vi "projekt.vi"() -> ()   [LabVIEW 2023]
doc: "Use this template to build a standard state machine design pattern. Each state executes code and determines which state to transition to. Contrast this design pattern with the User Interface Event Handler pattern, in which code executes in response to user actions. Contrast this design pattern also with the Queued Message Handler pattern, in which each message handling code can queue zero or more new messages.\nNote: This template does not contain the most recent programming guidelines recommended by National Instruments. For a complete, project-based implementation of the Standard State Machine pattern, use the Create Project dialog box instead of this template."
uses:
  projekt_stany.ctl
  <vilib>/DAQmx/read.llb/DAQmx Read (Digital 1D Bool 1Chan 1Samp).vi
  <vilib>/DAQmx/create/channels.llb/DAQmx Create Channel (DI-Digital Input).vi
  <vilib>/DAQmx/miscellaneous.llb/DAQmx Fill In Error Info.vi
panel:
  out "Nastepny Gracz":string
  in  "Wybierz Kto zaczyna":bool
  out "Wynik":string
  out "String 9":string
  out "String 8":string
  out "String 7":string
  out "String 6":string
  out "String 5":string
  out "String 4":string
  out "String 3":string
  out "String 2":string
  out "String":string
  in  "Stop":bool
  out "Kolumna":dbl
  out "Wiersz":dbl
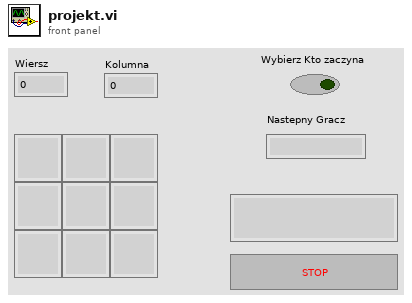
[diagram p1: front panel]
types:
  T1 = typedef "projekt_stany.ctl" = enum16{"Czysc", "Zapisz", "Wpisz", "Sprawdz", "Czytaj", "Initialize", "Stop"}
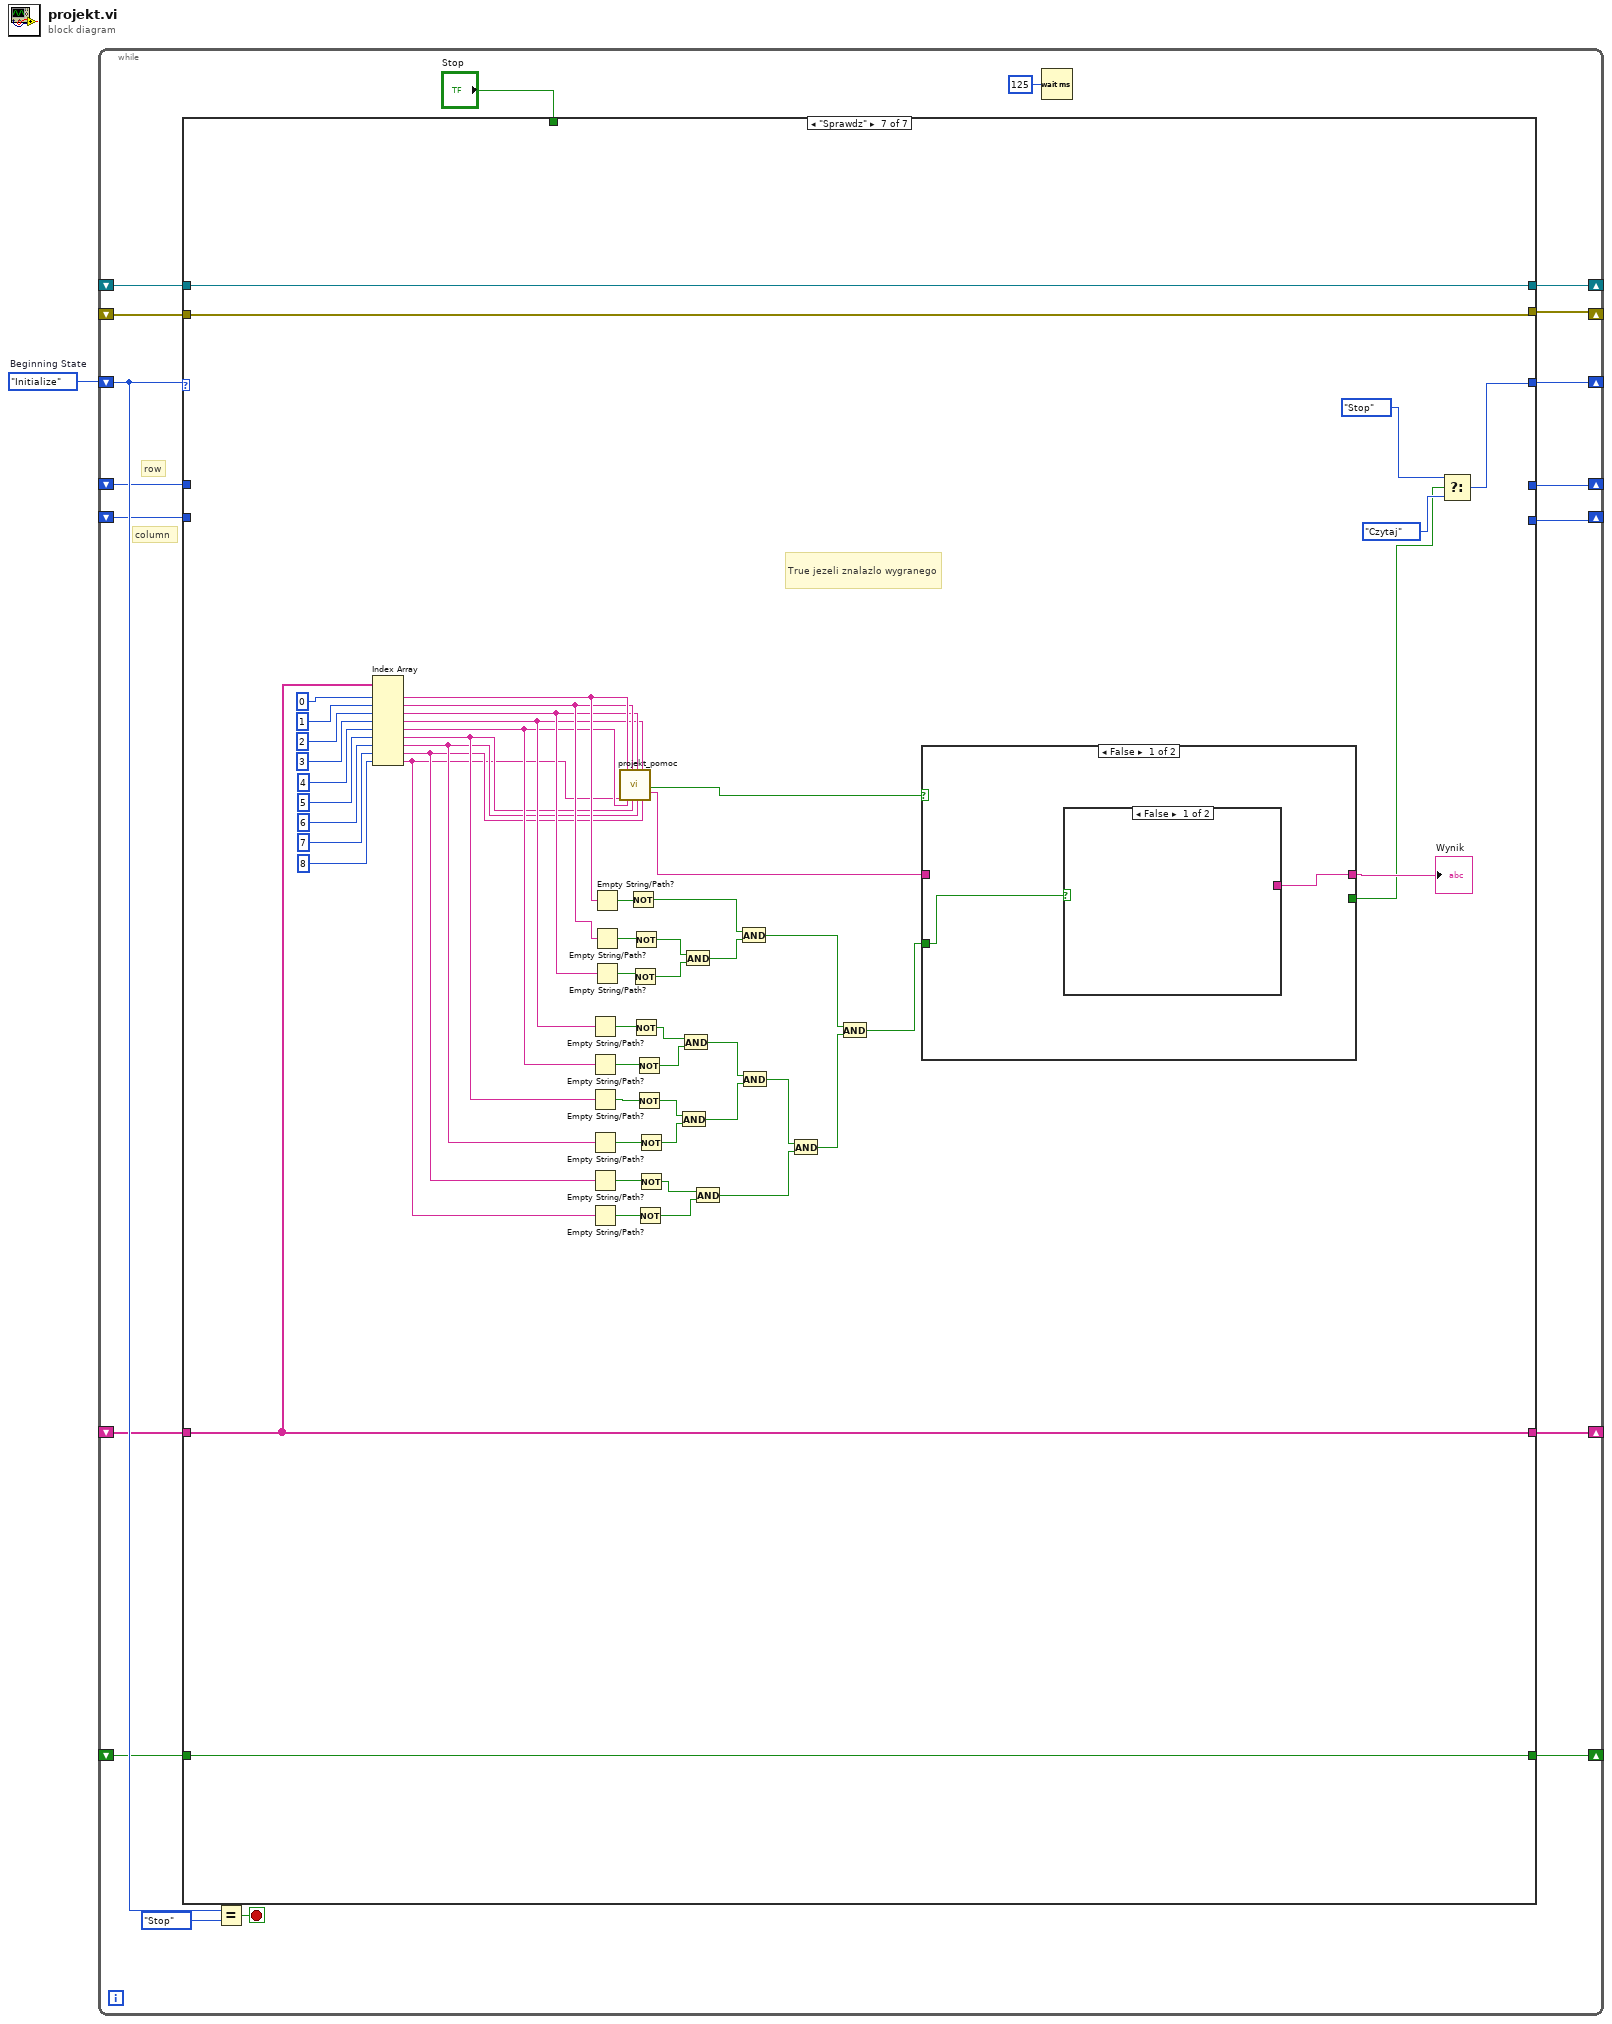
[diagram p0: block diagram]
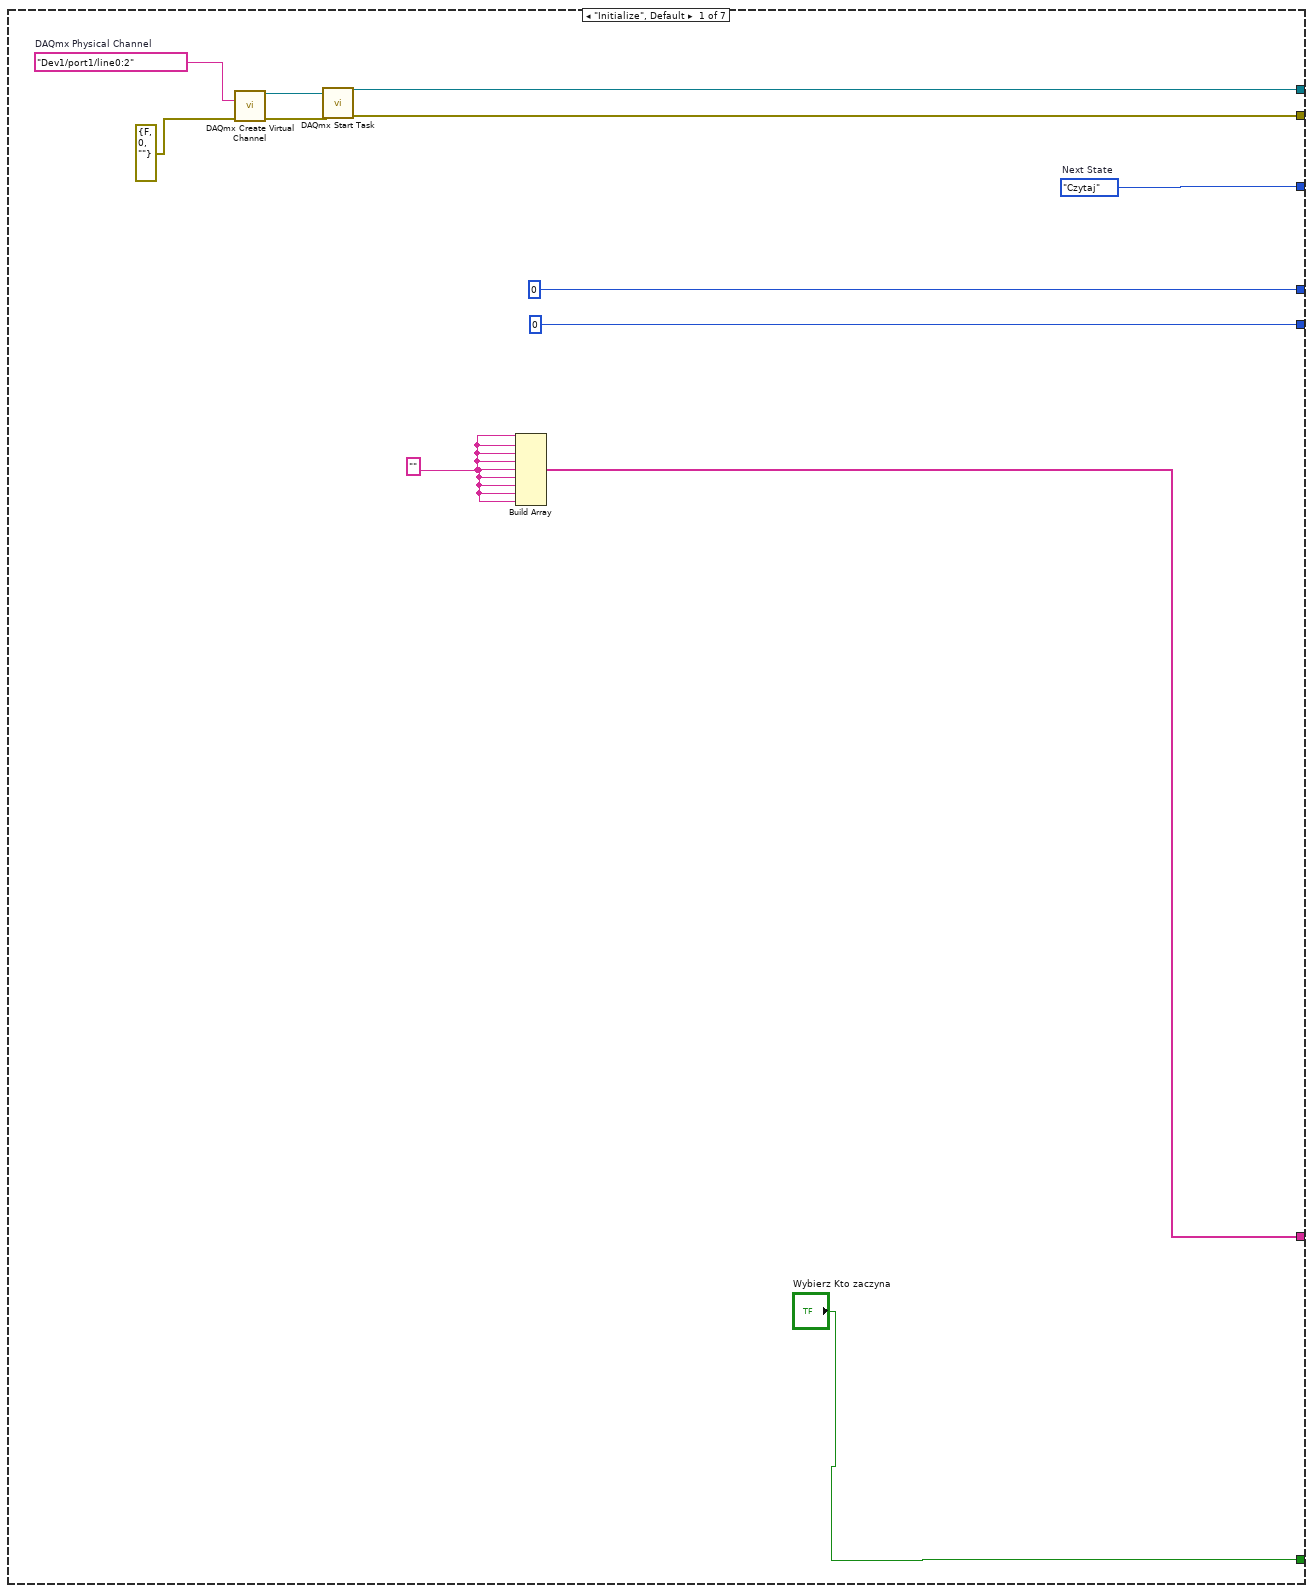
[diagram p2: hidden frame]
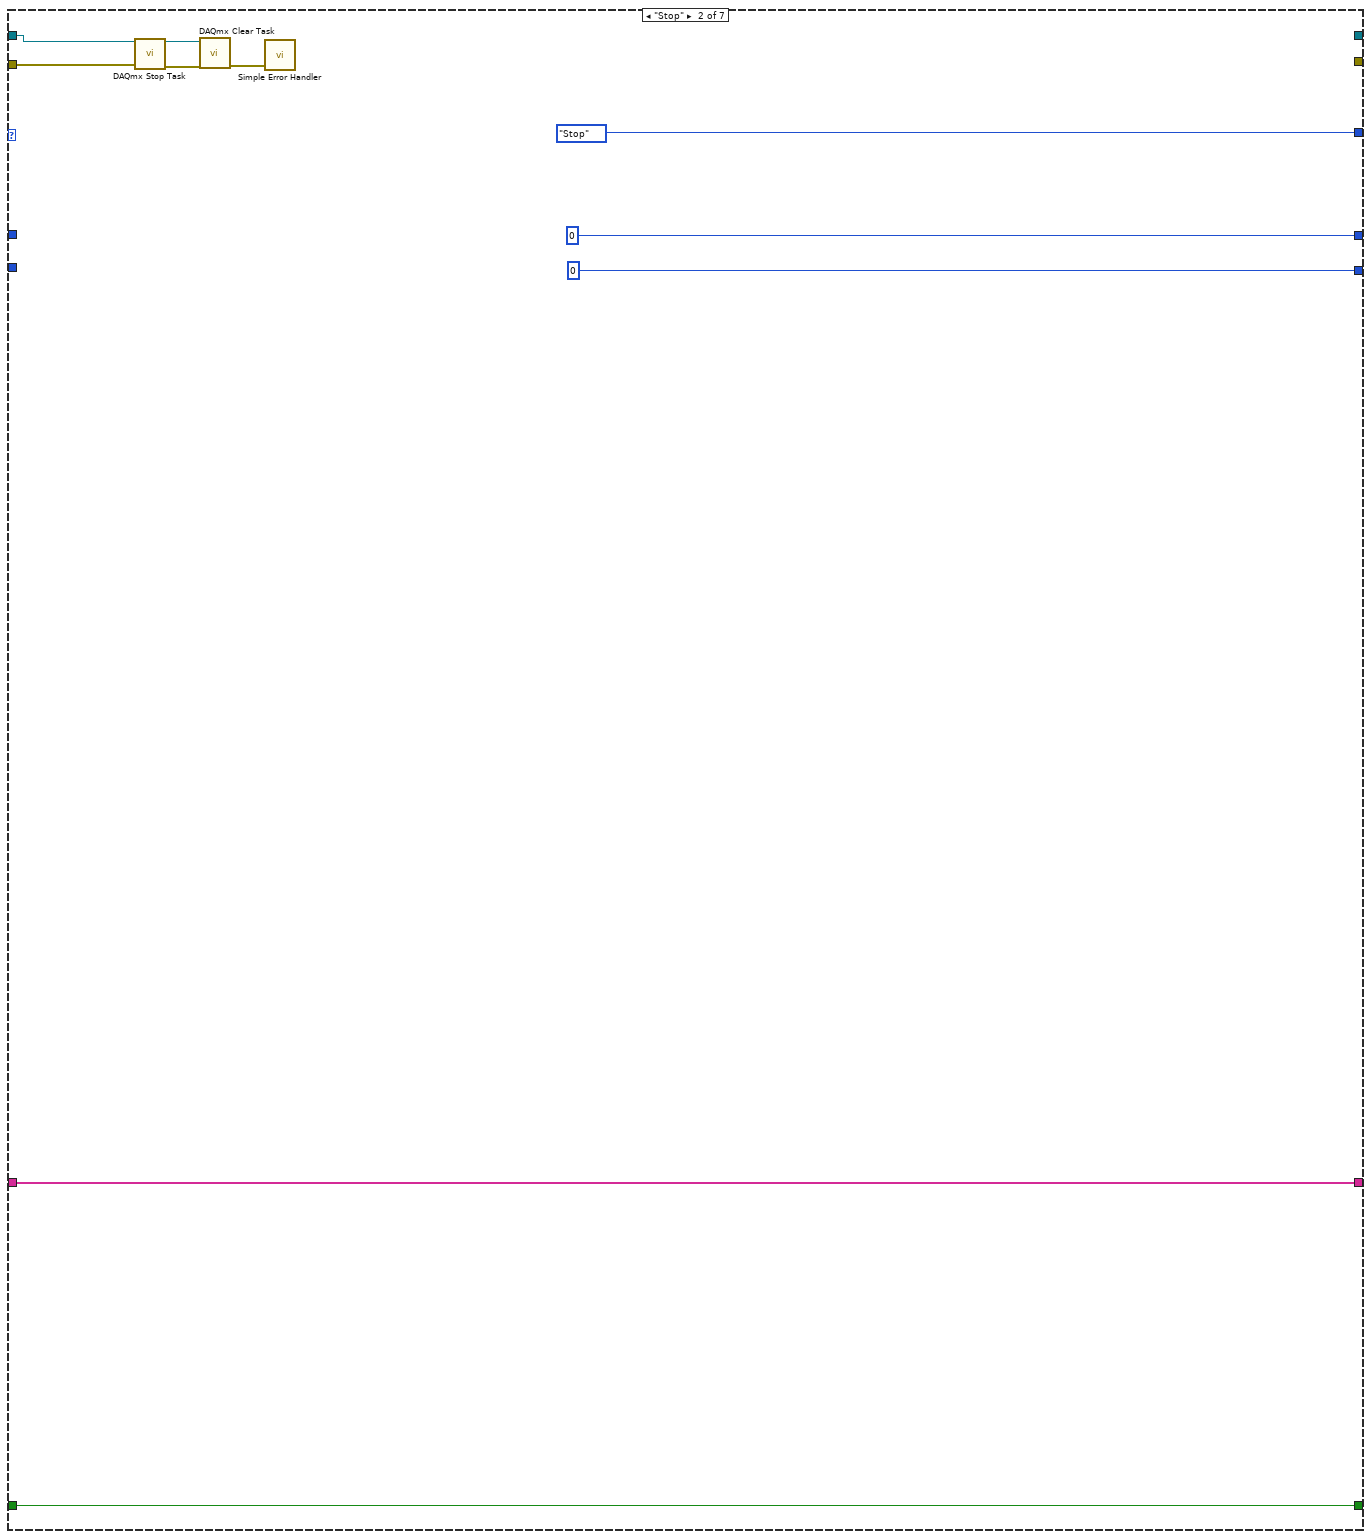
[diagram p3: hidden frame]
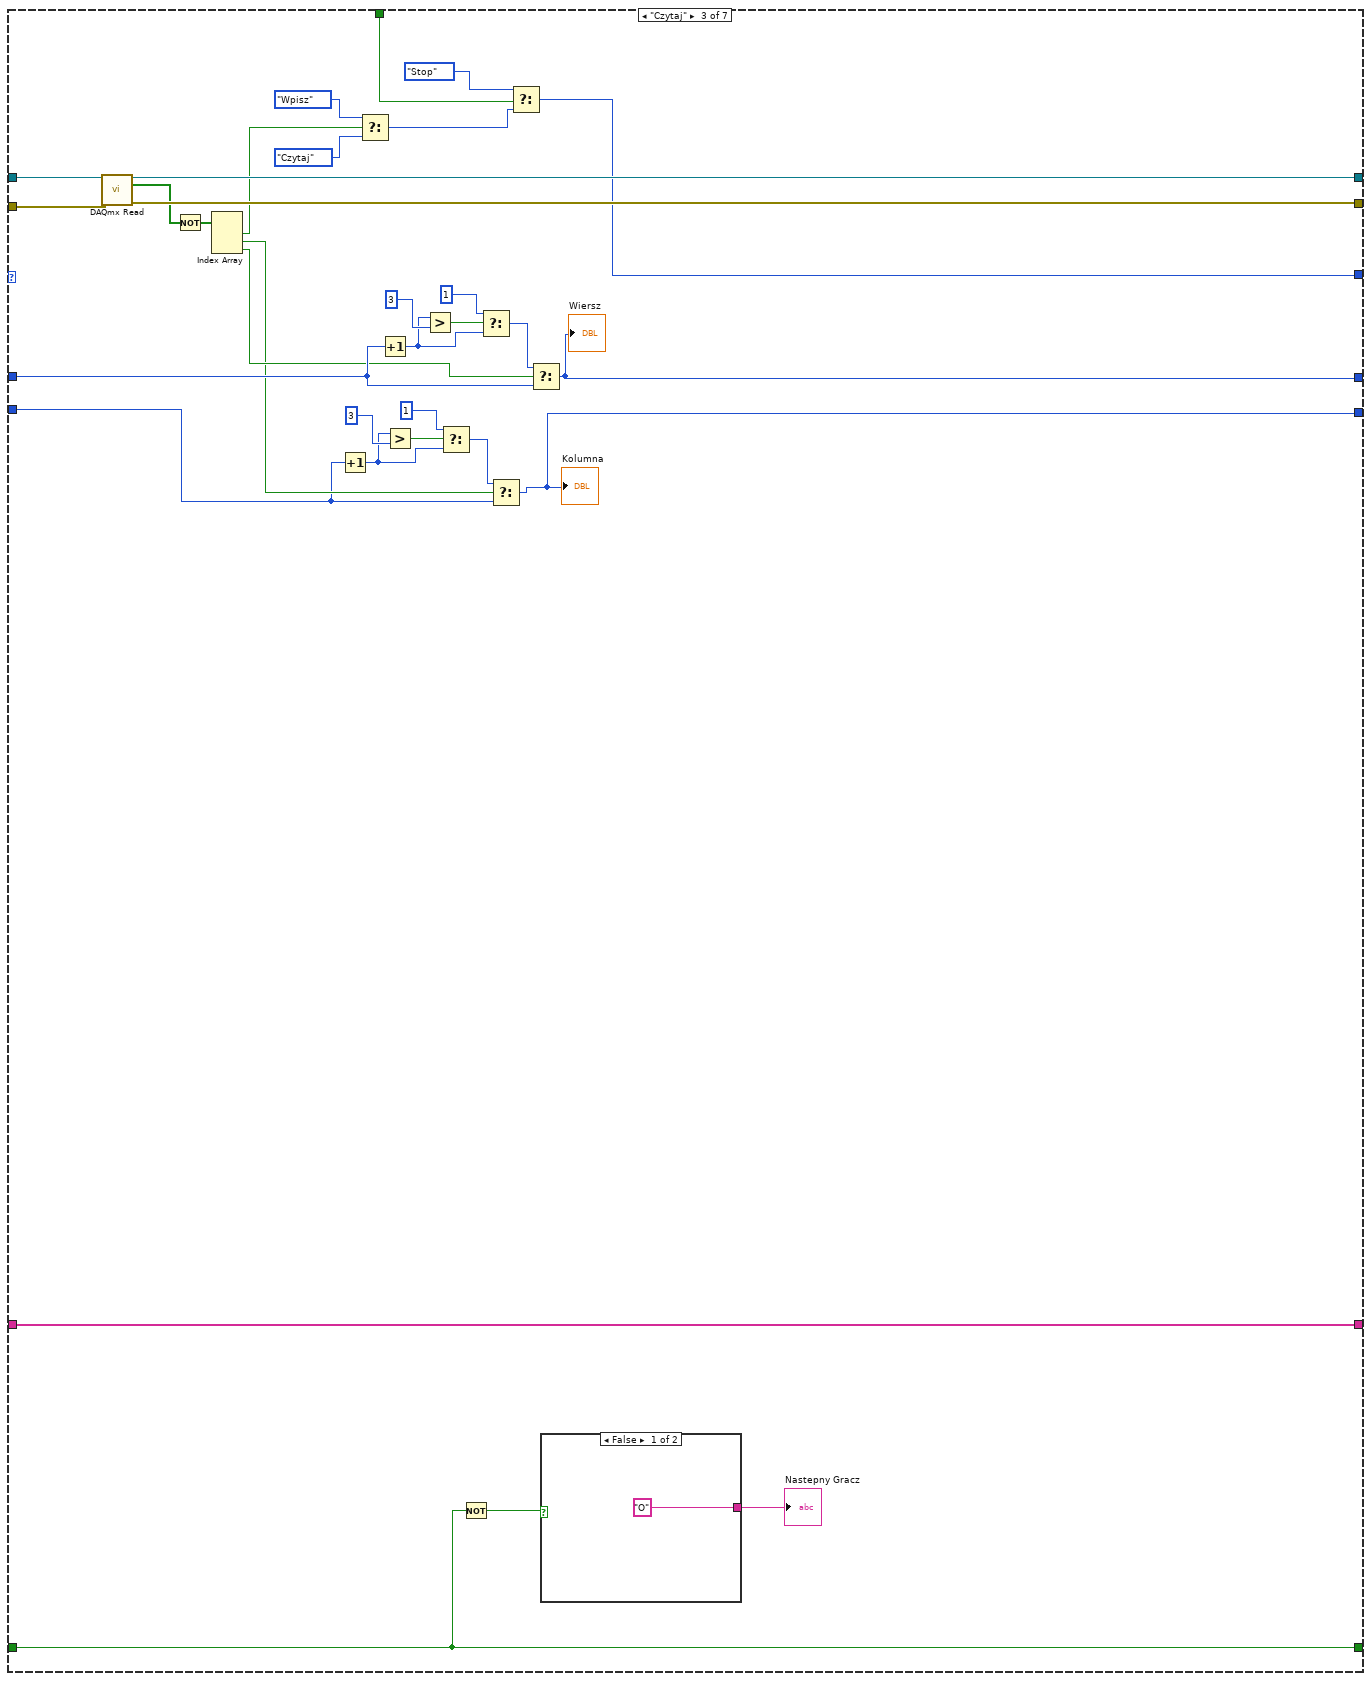
[diagram p4: hidden frame]
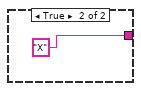
[diagram p5: hidden frame]
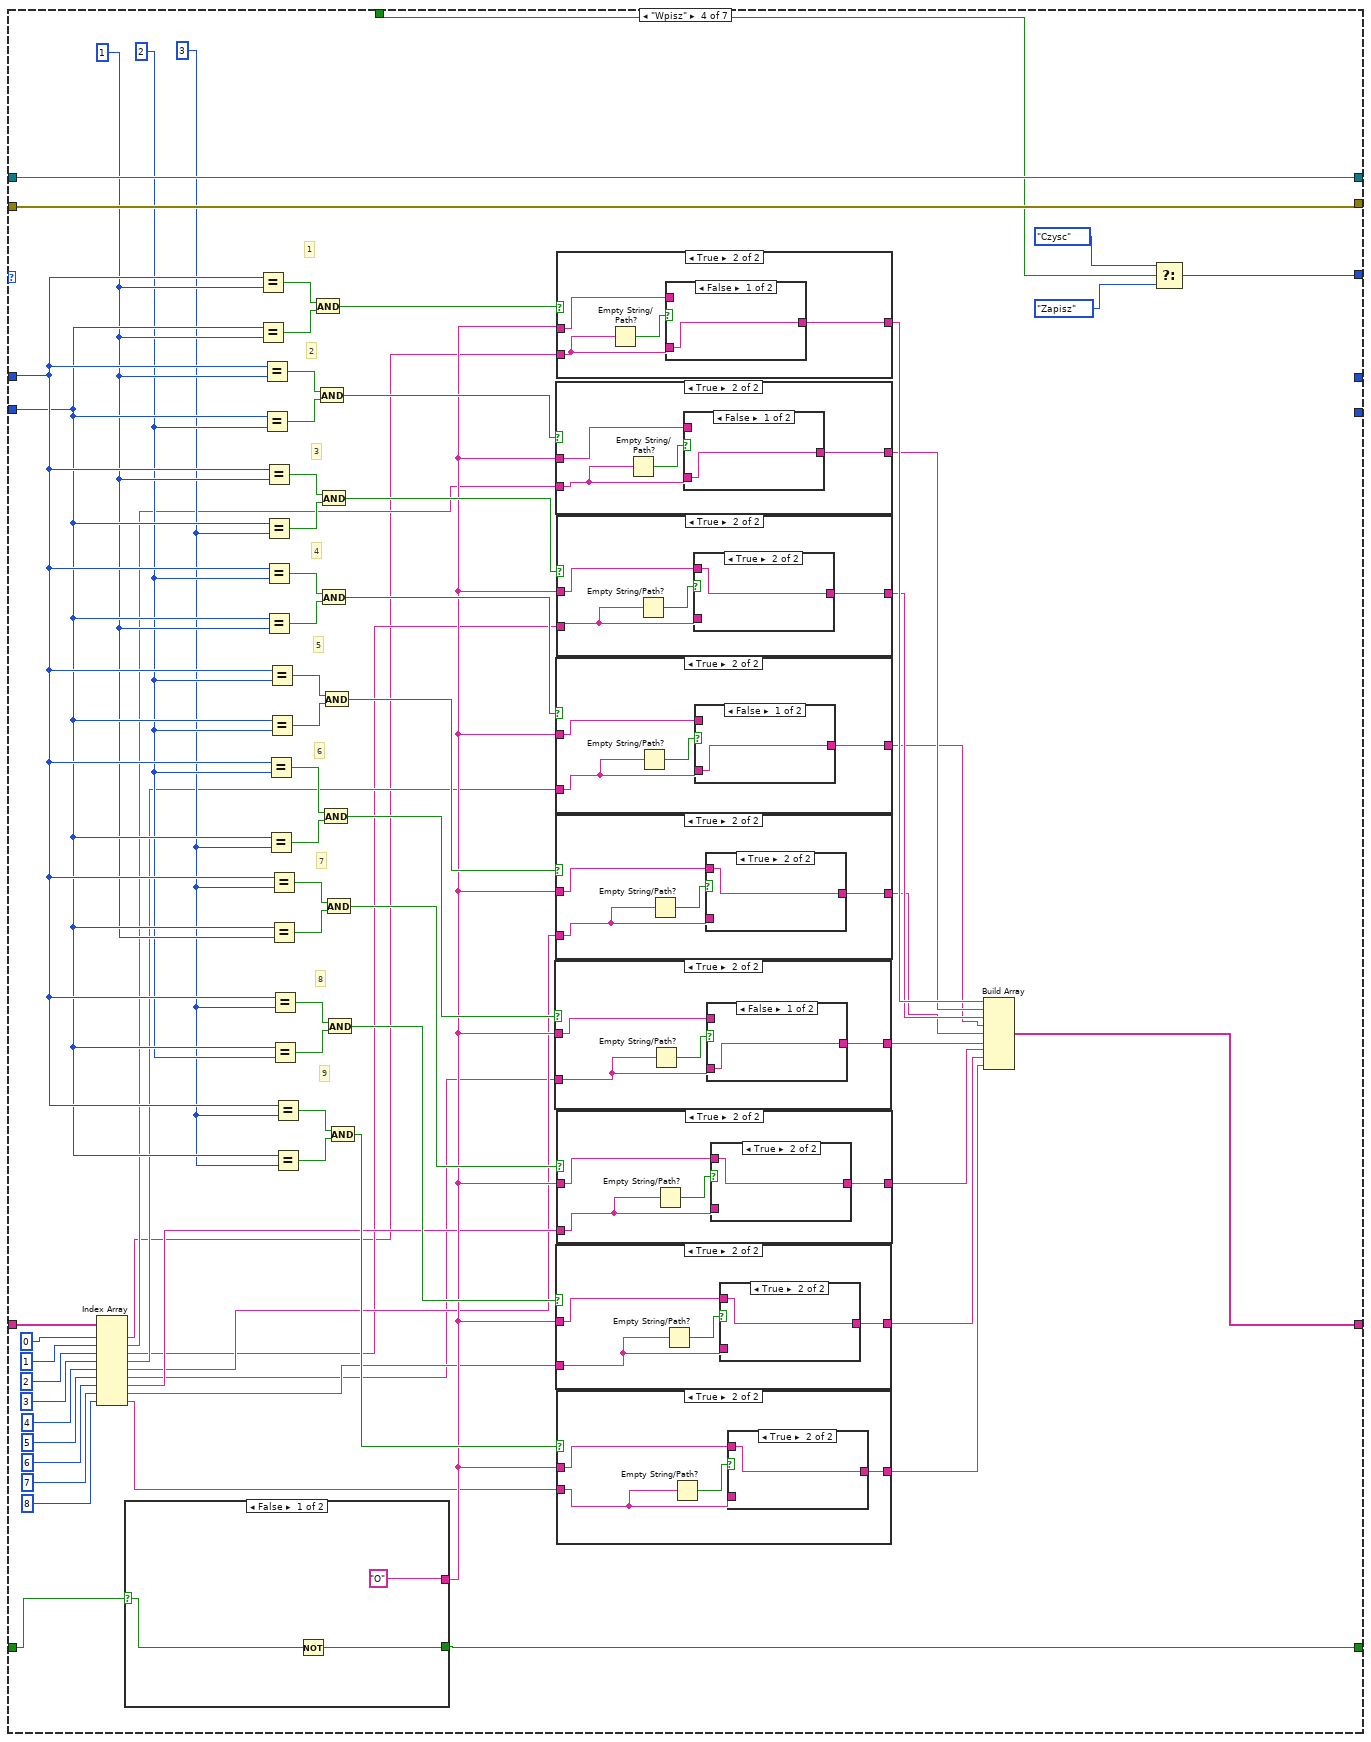
[diagram p6: hidden frame]
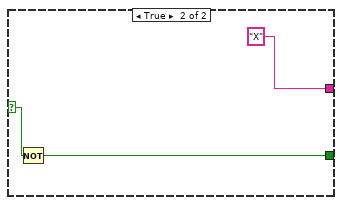
[diagram p7: hidden frame]
diagram:
  w1 = projekt_stany."Initialize"  # Beginning State
  n1 = while {
    shift-right: [w16] -> _
    shift-left: w1 -> [w17]
    shift-right: [w14] -> _
    shift-left: _ -> [w12]
    shift-right: [w13] -> _
    shift-left: _ -> [w11]
    shift-right: [w10] -> _
    shift-left: _ -> [w7]
    shift-right: [w9] -> _
    shift-left: _ -> [w8]
    shift-right: [w5] -> _
    shift-left: _ -> [w4]
    shift-right: [w2] -> _
    shift-left: _ -> [w3]
    stop <- w19 stop-if-true
    # "column"
    # "row"
    n2 = case shown="\"Sprawdz\"" w17 {
      tunnel: [w20 projekt_stany."Stop" ("Next State") w47 w111 w236 projekt_stany."Czysc" ("Next State") w288] -> w16
      tunnel: [w27 _ w72 w145 w240 w246 w301] -> w14
      tunnel: [w26 _ w71 w146 w241 w247 w302] -> w13
      tunnel: w12 -> [_ w39 w74 w145 w240 w246 w301]
      tunnel: w11 -> [_ w40 w73 w146 w241 w247 w302]
      tunnel: [0 0 w69 _ _ _ _] -> w10
      tunnel: [0 0 w55 _ _ _ _] -> w9
      tunnel: w8 -> [_ _ w53 w125 _ _ _]
      tunnel: w7 -> [_ _ w70 w126 _ _ _]
      tunnel: "Stop" -> [_ _ w46 w110 w235 _ _]
      tunnel: ["Wybierz Kto zaczyna" w33 w43 w77 w239 w245 w291] -> w5
      tunnel: w4 -> [_ w33 w43 w107 w239 w245 w291]
      tunnel: w3 -> [_ w32 w45 w106 w225 _ w287]
      tunnel: [w22 w32 w45 w79 w225 w243 w287] -> w2
      frame "Initialize", Default {
        w20 = projekt_stany."Czytaj"  # Next State
        w23 = ""
        w28 = tag "Dev1/port1/line0:2"  # DAQmx Physical Channel
        n3 = call-poly <vilib>:"DAQmx Create Virtual Channel.vi"("lines"=w28, "error in"=errorcluster {"status"=FALSE, "code"=0, "source"=""} ("error constant")) -> ("task out"=w29:refnum<k21>, "error out"=w30:errorcluster)  [unwired: 12 in]
        n4 = call <vilib>:"DAQmx Start Task.vi"("task/channels in"=w29, "error in"=w30) -> ("task out"=w26:refnum<k21>, "error out"=w27:errorcluster)  [unwired: 12 in]
        n5 = Build Array(w23, w23, w23, w23, w23, w23, w23, w23, w23) -> (w22:string[])
      }
      frame "Stop" {
        n6 = call <vilib>:"DAQmx Stop Task.vi"("task/channels in"=w40, "error in"=w39) -> ("task out"=w38:refnum<k21>, "error out"=w37:errorcluster)  [unwired: 12 in]
        n7 = call <vilib>:"DAQmx Clear Task.vi"("task in"=w38, "error in"=w37) -> ("error out"=w36:errorcluster)  [unwired: 13 in]
        n8 = call <vilib>:"Simple Error Handler.vi"("error in (no error)"=w36) -> ()  [unwired: 4 in, 5 out]
      }
      frame "Czytaj" {
        n9 = call-poly <vilib>:"DAQmx Read.vi"("task/channels in"=w73, "error in"=w74) -> ("task out"=w71:refnum<k21>, "data"=w63:bool[], "error out"=w72:errorcluster)  [unwired: 11 in]
        n10 = Not(x=w63) -> (.not. x?=w62:bool[])
        n11 = Index Array(array=w62) -> (element #1=w52:bool, element #2=w54:bool, element #3=w61:bool)  [unwired: 3 in]
        n12 = Increment(x=w53) -> (x+1=w57:i32)
        n13 = Select(t=projekt_stany."Wpisz" ("Next State"), s=w52, f=projekt_stany."Czytaj" ("Next State")) -> (s? t:f=w49:T1)
        n14 = Increment(x=w70) -> (x+1=w65:i32)
        n15 = Greater?(x=w57, y=3) -> (0:w59:bool)
        n16 = Greater?(x=w65, y=3) -> (0:w67:bool)
        n17 = Select(t=1, s=w59, f=w57) -> (s? t:f=w56:i32)
        n18 = Not(x=w43) -> (.not. x?=w44:bool)
        n19 = Select(t=1, s=w67, f=w65) -> (s? t:f=w64:i32)
        n20 = Select(t=w56, s=w54, f=w53) -> (s? t:f=w55:i32)
        "Kolumna" <- w55
        n21 = Select(t=projekt_stany."Stop" ("Next State"), s=w46, f=w49) -> (s? t:f=w47:T1)
        n22 = Select(t=w64, s=w61, f=w70) -> (s? t:f=w69:i32)
        "Wiersz" <- w69
        n23 = case shown="False" w44 {
          tunnel: ["O" "X"] -> w42
          frame False {
          }
          frame True {
          }
        }
        "Nastepny Gracz" <- w42
      }
      frame "Wpisz" {
        w122 = 3
        w123 = 2
        w124 = 1
        # "9"
        # "8"
        # "7"
        # "6"
        # "5"
        # "4"
        # "3"
        # "2"
        # "1"
        n24 = Index Array(array=w106, index #1=0, index #2=1, index #3=2, index #4=3, index #5=4, index #6=5, index #7=6, index #8=7, index #9=8) -> (element #1=w89:string, element #2=w90:string, element #3=w91:string, element #4=w92:string, element #5=w93:string, element #6=w78:string, element #7=w94:string, element #8=w95:string, element #9=w96:string)
        n25 = case shown="False" w107 {
          selector: w107 -> [w148 w151]
          tunnel: ["O" "X"] -> w108
          tunnel: [w147 w150] -> w77
          frame False {
            n26 = Not(x=w148) -> (.not. x?=w147:bool)
          }
          frame True {
            n27 = Not(x=w151) -> (.not. x?=w150:bool)
          }
        }
        n28 = Equal?(x=w126, y=w124) -> (x = y?=w144:bool)
        n29 = Equal?(x=w125, y=w124) -> (x = y?=w143:bool)
        n30 = Equal?(x=w126, y=w124) -> (x = y?=w142:bool)
        n31 = Equal?(x=w125, y=w123) -> (x = y?=w141:bool)
        n32 = Equal?(x=w126, y=w124) -> (x = y?=w140:bool)
        n33 = Equal?(x=w125, y=w122) -> (x = y?=w139:bool)
        n34 = Equal?(x=w126, y=w123) -> (x = y?=w138:bool)
        n35 = Equal?(x=w125, y=w124) -> (x = y?=w137:bool)
        n36 = Equal?(x=w126, y=w123) -> (x = y?=w134:bool)
        n37 = Equal?(x=w125, y=w122) -> (x = y?=w133:bool)
        n38 = Equal?(x=w126, y=w123) -> (x = y?=w136:bool)
        n39 = Equal?(x=w125, y=w123) -> (x = y?=w135:bool)
        n40 = Equal?(x=w126, y=w122) -> (x = y?=w132:bool)
        n41 = Equal?(x=w125, y=w124) -> (x = y?=w131:bool)
        n42 = Equal?(x=w126, y=w122) -> (x = y?=w130:bool)
        n43 = Equal?(x=w125, y=w123) -> (x = y?=w129:bool)
        n44 = Equal?(x=w126, y=w122) -> (x = y?=w128:bool)
        n45 = Equal?(x=w125, y=w122) -> (x = y?=w127:bool)
        n46 = And(x=w144, y=w143) -> (x .and. y?=w109:bool)
        n47 = And(x=w142, y=w141) -> (x .and. y?=w121:bool)
        n48 = And(x=w140, y=w139) -> (x .and. y?=w120:bool)
        n49 = And(x=w138, y=w137) -> (x .and. y?=w119:bool)
        n50 = And(x=w134, y=w133) -> (x .and. y?=w117:bool)
        n51 = And(x=w136, y=w135) -> (x .and. y?=w118:bool)
        n52 = And(x=w132, y=w131) -> (x .and. y?=w116:bool)
        n53 = And(x=w130, y=w129) -> (x .and. y?=w115:bool)
        n54 = And(x=w128, y=w127) -> (x .and. y?=w114:bool)
        n55 = case shown="True" w117 {
          tunnel: w108 -> [_ w176]
          tunnel: [w174 w177] -> w83
          tunnel: w78 -> [w174 w175]
          frame False {
          }
          frame True {
            n56 = Empty String/Path?(string/path=w175) -> (empty?=w178:bool)
            n57 = case shown="False" w178 {
              tunnel: w176 -> [_ w180]
              tunnel: w175 -> [w179 _]
              tunnel: [w179 w180] -> w177
              frame False {
              }
              frame True {
              }
            }
          }
        }
        n58 = case shown="True" w121 {
          tunnel: w108 -> [_ w205]
          tunnel: w90 -> [w202 w204]
          tunnel: [w202 w203] -> w87
          frame False {
          }
          frame True {
            n59 = Empty String/Path?(string/path=w204) -> (empty?=w206:bool)
            n60 = case shown="False" w206 {
              tunnel: w205 -> [_ w208]
              tunnel: w204 -> [w207 _]
              tunnel: [w207 w208] -> w203
              frame False {
              }
              frame True {
              }
            }
          }
        }
        n61 = case shown="True" w119 {
          tunnel: w108 -> [_ w191]
          tunnel: w92 -> [w188 w190]
          tunnel: [w188 w189] -> w85
          frame False {
          }
          frame True {
            n62 = Empty String/Path?(string/path=w190) -> (empty?=w192:bool)
            n63 = case shown="False" w192 {
              tunnel: w191 -> [_ w194]
              tunnel: w190 -> [w193 _]
              tunnel: [w193 w194] -> w189
              frame False {
              }
              frame True {
              }
            }
          }
        }
        n64 = case shown="True" w118 {
          tunnel: w108 -> [_ w184]
          tunnel: w93 -> [w181 w183]
          tunnel: [w181 w182] -> w84
          frame False {
          }
          frame True {
            n65 = Empty String/Path?(string/path=w183) -> (empty?=w185:bool)
            n66 = case shown="True" w185 {
              tunnel: w184 -> [_ w187]
              tunnel: w183 -> [w186 _]
              tunnel: [w186 w187] -> w182
              frame False {
              }
              frame True {
              }
            }
          }
        }
        n67 = case shown="True" w115 {
          tunnel: w108 -> [_ w163]
          tunnel: w95 -> [w160 w162]
          tunnel: [w160 w161] -> w81
          frame False {
          }
          frame True {
            n68 = Empty String/Path?(string/path=w162) -> (empty?=w164:bool)
            n69 = case shown="True" w164 {
              tunnel: w163 -> [_ w166]
              tunnel: w162 -> [w165 _]
              tunnel: [w165 w166] -> w161
              frame False {
              }
              frame True {
              }
            }
          }
        }
        n70 = case shown="True" w109 {
          tunnel: w108 -> [_ w212]
          tunnel: w89 -> [w209 w211]
          tunnel: [w209 w210] -> w88
          frame False {
          }
          frame True {
            n71 = Empty String/Path?(string/path=w211) -> (empty?=w213:bool)
            n72 = case shown="False" w213 {
              tunnel: w212 -> [_ w215]
              tunnel: w211 -> [w214 _]
              tunnel: [w214 w215] -> w210
              frame False {
              }
              frame True {
              }
            }
          }
        }
        n73 = case shown="True" w120 {
          tunnel: w108 -> [_ w197]
          tunnel: w91 -> [w195 w198]
          tunnel: [w195 w196] -> w86
          frame False {
          }
          frame True {
            n74 = Empty String/Path?(string/path=w198) -> (empty?=w199:bool)
            n75 = case shown="True" w199 {
              tunnel: w197 -> [_ w201]
              tunnel: w198 -> [w200 _]
              tunnel: [w200 w201] -> w196
              frame False {
              }
              frame True {
              }
            }
          }
        }
        n76 = case shown="True" w116 {
          tunnel: w108 -> [_ w170]
          tunnel: w94 -> [w167 w169]
          tunnel: [w167 w168] -> w82
          frame False {
          }
          frame True {
            n77 = Empty String/Path?(string/path=w169) -> (empty?=w171:bool)
            n78 = case shown="True" w171 {
              tunnel: w170 -> [_ w173]
              tunnel: w169 -> [w172 _]
              tunnel: [w172 w173] -> w168
              frame False {
              }
              frame True {
              }
            }
          }
        }
        n79 = case shown="True" w114 {
          tunnel: w108 -> [_ w156]
          tunnel: w96 -> [w153 w155]
          tunnel: [w153 w154] -> w80
          frame False {
          }
          frame True {
            n80 = Empty String/Path?(string/path=w155) -> (empty?=w157:bool)
            n81 = case shown="True" w157 {
              tunnel: w156 -> [_ w159]
              tunnel: w155 -> [w158 _]
              tunnel: [w158 w159] -> w154
              frame False {
              }
              frame True {
              }
            }
          }
        }
        n82 = Build Array(w88, w87, w86, w85, w84, w83, w82, w81, w80) -> (w79:string[])
        n83 = Select(t=projekt_stany."Czysc" ("Next State"), s=w110, f=projekt_stany."Zapisz" ("Next State")) -> (s? t:f=w111:T1)
      }
      frame "Zapisz" {
        n84 = Index Array(array=w225, index #1=0, index #2=1, index #3=2, index #4=3, index #5=4, index #6=5, index #7=6, index #8=7, index #9=8) -> (element #1=→"String":string, element #2=→"String 2":string, element #3=→"String 3":string, element #4=→"String 4":string, element #5=→"String 5":string, element #6=→"String 6":string, element #7=→"String 7":string, element #8=→"String 8":string, element #9=→"String 9":string)
        n85 = Select(t=projekt_stany."Czysc" ("Next State"), s=w235, f=projekt_stany."Sprawdz" ("Next State")) -> (s? t:f=w236:T1)
      }
      frame "Czysc" {
        w244 = ""
        n86 = Build Array(w244, w244, w244, w244, w244, w244, w244, w244, w244) -> (w243:string[])
      }
      frame "Sprawdz" {
        # "True jezeli znalazlo wygranego"
        n87 = Index Array(array=w287, index #1=0, index #2=1, index #3=2, index #4=3, index #5=4, index #6=5, index #7=6, index #8=7, index #9=8) -> (element #1=w286:string, element #2=w285:string, element #3=w284:string, element #4=w283:string, element #5=w282:string, element #6=w281:string, element #7=w280:string, element #8=w279:string, element #9=w278:string)
        n88 = Empty String/Path?(string/path=w283) -> (empty?=w272:bool)
        n89 = Empty String/Path?(string/path=w282) -> (empty?=w273:bool)
        n90 = Empty String/Path?(string/path=w281) -> (empty?=w274:bool)
        n91 = Empty String/Path?(string/path=w280) -> (empty?=w275:bool)
        n92 = Empty String/Path?(string/path=w279) -> (empty?=w276:bool)
        n93 = Empty String/Path?(string/path=w278) -> (empty?=w277:bool)
        n94 = Empty String/Path?(string/path=w286) -> (empty?=w269:bool)
        n95 = Empty String/Path?(string/path=w285) -> (empty?=w270:bool)
        n96 = Empty String/Path?(string/path=w284) -> (empty?=w271:bool)
        n97 = call "projekt_pomoc.vi"("String 9"=w278, "String"=w286, "String 5"=w282, "String 2"=w285, "String 6"=w281, "String 3"=w284, "String 7"=w280, "String 4"=w283, "String 8"=w279) -> ("x .or. y?"=w249:bool, "String 10"=w252:string)  [unwired: 9 in]
        n98 = Not(x=w269) -> (.not. x?=w260:bool)
        n99 = Not(x=w271) -> (.not. x?=w262:bool)
        n100 = Not(x=w270) -> (.not. x?=w261:bool)
        n101 = Not(x=w272) -> (.not. x?=w263:bool)
        n102 = Not(x=w273) -> (.not. x?=w264:bool)
        n103 = Not(x=w274) -> (.not. x?=w265:bool)
        n104 = Not(x=w277) -> (.not. x?=w268:bool)
        n105 = Not(x=w275) -> (.not. x?=w266:bool)
        n106 = Not(x=w276) -> (.not. x?=w267:bool)
        n107 = And(x=w265, y=w266) -> (x .and. y?=w258:bool)
        n108 = And(x=w263, y=w264) -> (x .and. y?=w257:bool)
        n109 = And(x=w261, y=w262) -> (x .and. y?=w259:bool)
        n110 = And(x=w267, y=w268) -> (x .and. y?=w256:bool)
        n111 = And(x=w260, y=w259) -> (x .and. y?=w253:bool)
        n112 = And(x=w257, y=w258) -> (x .and. y?=w255:bool)
        n113 = And(x=w255, y=w256) -> (x .and. y?=w254:bool)
        n114 = And(x=w253, y=w254) -> (x .and. y?=w250:bool)
        n115 = case shown="False" w249 {
          selector: w249 -> [_ w309]
          tunnel: w252 -> [_ w308]
          tunnel: [w303 w307] -> w251
          tunnel: w250 -> [w304 _]
          tunnel: [_ w306] -> w248
          frame False {
            n116 = case shown="False" w304 {
              tunnel: [_ "REMIS"] -> w303
              frame False {
              }
              frame True {
              }
            }
          }
          frame True {
            n117 = case shown="False" w309 {
              selector: w309 -> [_ w310]
              tunnel: w308 -> [_ w311]
              tunnel: [_ w311] -> w307
              tunnel: [_ w310] -> w306
              frame False {
              }
              frame True {
              }
            }
          }
        }
        "Wynik" <- w251
        n118 = Select(t=projekt_stany."Stop" ("Next State"), s=w248, f=projekt_stany."Czytaj" ("Next State")) -> (s? t:f=w288:T1)
      }
    }
    n119 = Equal?(x=w17, y=projekt_stany."Stop" ("States")) -> (x = y?=w19:bool)
    n120 = Wait (ms)(milliseconds to wait=u32 125) -> ()  [unwired: 1 out]
  }
